vi "TDT-Close Tank.vi"(0 "Data":T2={"TTankX"=refnum, "TDevAccX"=refnum, "LastTime"=0.0, "error"={"status"=FALSE, "code"=0, "source"=""}, "Block Name"="", "Circuit Tag"="", "Tank Name"="", "NumTicks"=0, "LastTick"=0.0, "Idle?"=FALSE, "Wait (ms)"=1000, "LastArtf"=0.0, "LastTosc"=0.0}, 7 "Mode":T1, 11 "error in (no error)":errorcluster) -> (6 "TankName":string, 8 "Block Name":string, 15 "error out":errorcluster)   [LabVIEW 2015]
uses:
  TDT Interface Data.ctl
  TDT-Sys Mode Enum.ctl
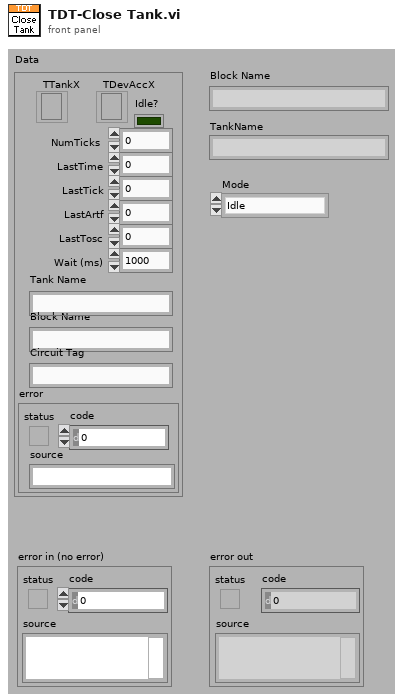
[diagram p1: front panel]
types:
  T1 = typedef "TDT-Sys Mode Enum.ctl" = enum16{"Idle", "Standby", "Preview", "Record"}
  T2 = typedef "TDT Interface Data.ctl" = cluster{"TTankX":refnum<k7>, "TDevAccX":refnum<k7>, "LastTime":dbl, "error":errorcluster, "Block Name":string, "Circuit Tag":string, "Tank Name":string, "NumTicks":i32, "LastTick":dbl, "Idle?":bool, "Wait (ms)":u32, "LastArtf":dbl, "LastTosc":dbl}
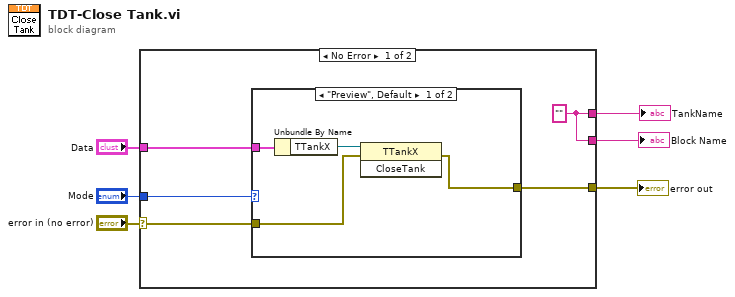
[diagram p0: block diagram]
diagram:
  n1 = case shown="No Error" "error in (no error)" {
    selector: "error in (no error)" -> [w9 w17]
    tunnel: [w11 w17] -> w5
    tunnel: "Data" -> [w10 _]
    tunnel: [w7 _] -> w3
    tunnel: "Mode" -> [w8 _]
    tunnel: [w7 _] -> w1
    frame No Error {
      w7 = "" ("BlockName")
      n2 = case shown="\"Preview\", Default" w8 {
        tunnel: [w12 w16] -> w11
        tunnel: w10 -> [w15 _]
        tunnel: w9 -> [w13 w16]
        frame "Preview", Default {
          n3 = Unbundle By Name(w15) -> ("TTankX"=w14:refnum<k7>)
          n4 = invoke class="TTankX" method="CloseTank"(reference=w14, error in=w13) -> (error out=w12:errorcluster)  [unwired: 1 in, 2 out]
        }
        frame "Record" {
        }
      }
    }
    frame Error {
    }
  }
  "error out" <- w5
  "Block Name" <- w3
  "TankName" <- w1
